vi "Read Buffer Size.vi"(11 "Template in":refnum<class "Template.lvclass">) -> (3 "DVR Pool Size":i32)   [LabVIEW 2020, in "Template.lvlib" / "Template.lvclass"]
doc: "Returns the standard buffer size for this actor"
uses:
  Template.lvclass
  Template.lvclass/Template.ctl
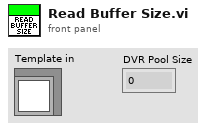
[diagram p1: front panel]
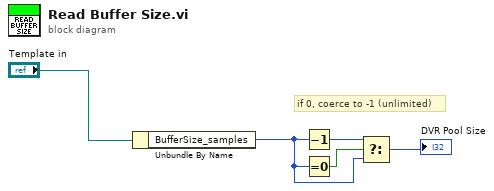
[diagram p0: block diagram]
diagram:
  # "if 0, coerce to -1 (unlimited)"
  n1 = Unbundle By Name("Template in") -> ("BufferSize_samples"=w2:i32)
  n2 = Decrement(x=w2) -> (x-1=w3:i32)
  n3 = Equal To 0?(x=w2) -> (x = 0?=w4:bool)
  n4 = Select(t=w3, s=w4, f=w2) -> (s? t:f=→"DVR Pool Size":i32)
